vi "New.vi"(7 "Table of Contents?":bool, 8 "error in (no error)":errorcluster, 9 "Default topic":string, 10 "Title":string, 11 "Base Path":path) -> (0 "error out":errorcluster, 3 "CHM Generator out":refnum<class "CHM Generator.lvclass">)   [LabVIEW 2015, in "CHM Generator.lvclass"]
uses:
  CHM Generator.lvclass
  CHM Generator.lvclass/CHM Generator.ctl
  Keyed Value Tree/Keyed Value Tree.lvclass
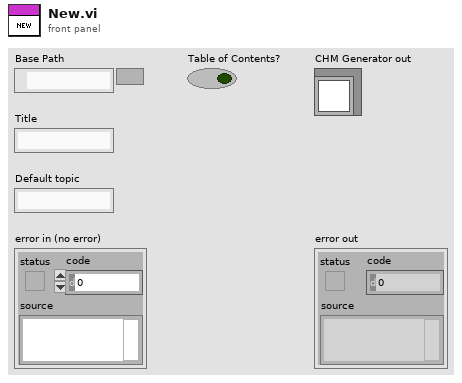
[diagram p1: front panel]
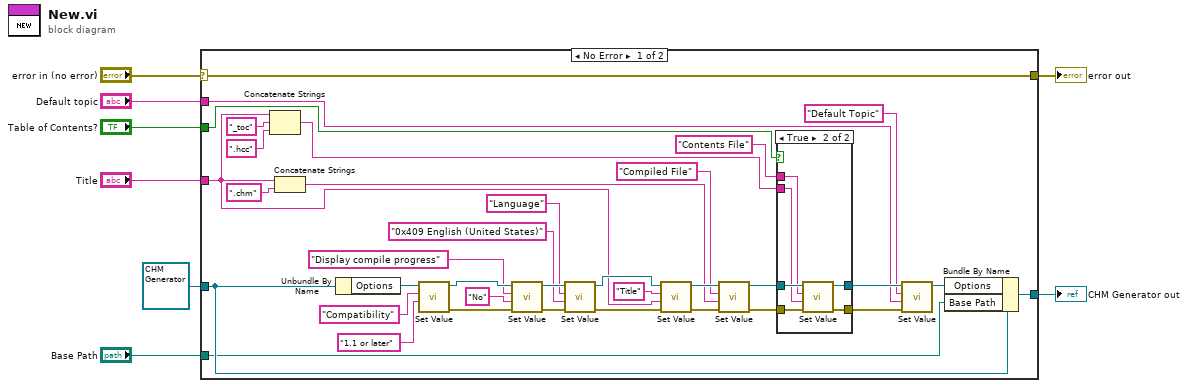
[diagram p0: block diagram]
diagram:
  n1 = case shown="No Error" "error in (no error)" {
    selector: "error in (no error)" -> [w44 w54]
    tunnel: [w44 w54] -> w7
    tunnel: [w17 w53] -> w5
    tunnel: refnum<class "CHM Generator.lvclass"> refnum ("CHM Generator in") -> [w19 w53]
    tunnel: "Default topic" -> [w20 _]
    tunnel: "Title" -> [w13 _]
    tunnel: "Base Path" -> [w11 _]
    tunnel: "Table of Contents?" -> [w9 _]
    frame No Error {
      n2 = Concatenate Strings(w13, "_toc" ("string"), ".hcc" ("string")) -> (w10:string)
      n3 = Concatenate Strings(w13, ".chm" ("string")) -> (w15:string)
      n4 = Unbundle By Name(w19) -> ("Options"=w41:refnum<class "Keyed Value Tree.lvclass">)
      n5 = call-dynamic "Set Value.vi"("value"="1.1 or later", "name"="Compatibility", "Keyed Value Tree in"=w41) -> ("error out"=w39:errorcluster, "Keyed Value Tree out"=w40:refnum<class "Keyed Value Tree.lvclass">)  [unwired: 6 in, 1 out]
      n6 = call-dynamic "Set Value.vi"("error in (no error)"=w39, "value"="No", "name"="Display compile progress", "Keyed Value Tree in"=w40) -> ("error out"=w36:errorcluster, "Keyed Value Tree out"=w35:refnum<class "Keyed Value Tree.lvclass">)  [unwired: 5 in, 1 out]
      n7 = call-dynamic "Set Value.vi"("error in (no error)"=w36, "value"="0x409 English (United States)", "name"="Language", "Keyed Value Tree in"=w35) -> ("error out"=w31:errorcluster, "Keyed Value Tree out"=w32:refnum<class "Keyed Value Tree.lvclass">)  [unwired: 5 in, 1 out]
      n8 = call-dynamic "Set Value.vi"("error in (no error)"=w31, "value"=w13, "name"="Title", "Keyed Value Tree in"=w32) -> ("error out"=w30:errorcluster, "Keyed Value Tree out"=w29:refnum<class "Keyed Value Tree.lvclass">)  [unwired: 5 in, 1 out]
      n9 = call-dynamic "Set Value.vi"("error in (no error)"=w30, "value"=w15, "name"="Compiled File", "Keyed Value Tree in"=w29) -> ("error out"=w28:errorcluster, "Keyed Value Tree out"=w27:refnum<class "Keyed Value Tree.lvclass">)  [unwired: 5 in, 1 out]
      n10 = case shown="True" w9 {
        tunnel: w28 -> [w45 w52]
        tunnel: w27 -> [w46 w51]
        tunnel: [w45 w50] -> w26
        tunnel: [w46 w49] -> w25
        tunnel: "Contents File" ("name") -> [_ w48]
        tunnel: w10 -> [_ w47]
        frame False {
        }
        frame True {
          n11 = call-dynamic "Set Value.vi"("error in (no error)"=w52, "value"=w47, "name"=w48, "Keyed Value Tree in"=w51) -> ("error out"=w50:errorcluster, "Keyed Value Tree out"=w49:refnum<class "Keyed Value Tree.lvclass">)  [unwired: 5 in, 1 out]
        }
      }
      n12 = call-dynamic "Set Value.vi"("error in (no error)"=w26, "value"=w20, "name"="Default Topic", "Keyed Value Tree in"=w25) -> ("Keyed Value Tree out"=w18:refnum<class "Keyed Value Tree.lvclass">)  [unwired: 5 in, 2 out]
      n13 = Bundle By Name(cluster=w19, "Options"=w18, "Base Path"=w11) -> (w17:refnum<class "CHM Generator.lvclass">)
    }
    frame Error {
    }
  }
  "error out" <- w7
  "CHM Generator out" <- w5
